vi "Calculate Pixel Reciprocals.vi"(11 "Sorted Triangle":T1={"Top Vertex"={"Position"={"x"=0.0, "y"=0.0, "z"=0.0}, "UV"={"u"=0.0, "v"=0.0}, "Colour"=12517256}, "Mid Vertex"={"Position"={"x"=0.0, "y"=0.0, "z"=0.0}, "UV"={"u"=0.0, "v"=0.0}, "Colour"=12517256}, "Bottom Vertex"={"Position"={"x"=0.0, "y"=0.0, "z"=0.0}, "UV"={"u"=0.0, "v"=0.0}, "Colour"=12517256}, "Alpha"=0.0, "Alpha Blending Enabled"=FALSE, "Colour"=0, "Material"={"Diffuse Colour"=0, "Texture"={"Pixels"=refnum, "Size"={"Width"=0, "Height"=0}}}} {"Bottom Vertex"."UV"."v" min=0 max=1 step=0.1; "Bottom Vertex"."UV"."u" min=0 max=1 step=0.1; "Mid Vertex"."UV"."v" min=0 max=1 step=0.1; "Mid Vertex"."UV"."u" min=0 max=1 step=0.1; "Top Vertex"."UV"."v" min=0 max=1 step=0.1; "Top Vertex"."UV"."u" min=0 max=1 step=0.1}) -> (3 "Columns Pixels Per Row":T8)   [LabVIEW 2020, in "Raster (FPGA).lvlib"]
uses:
  Raster (FPGA).lvlib
  Reciprocals.ctl
  Libraries/3D/Vector 3D.ctl
  Libraries/3D/3D.lvlib
  Libraries/3D/Vertex.ctl
  Libraries/3D/Triangle (Sorted).ctl
  Libraries/3D/Material.ctl
  Libraries/Raster/UV.ctl
  Libraries/Raster/Raster.lvlib
  Libraries/Raster/Rectangle Dimensions.ctl
  Libraries/Raster/Texture.ctl
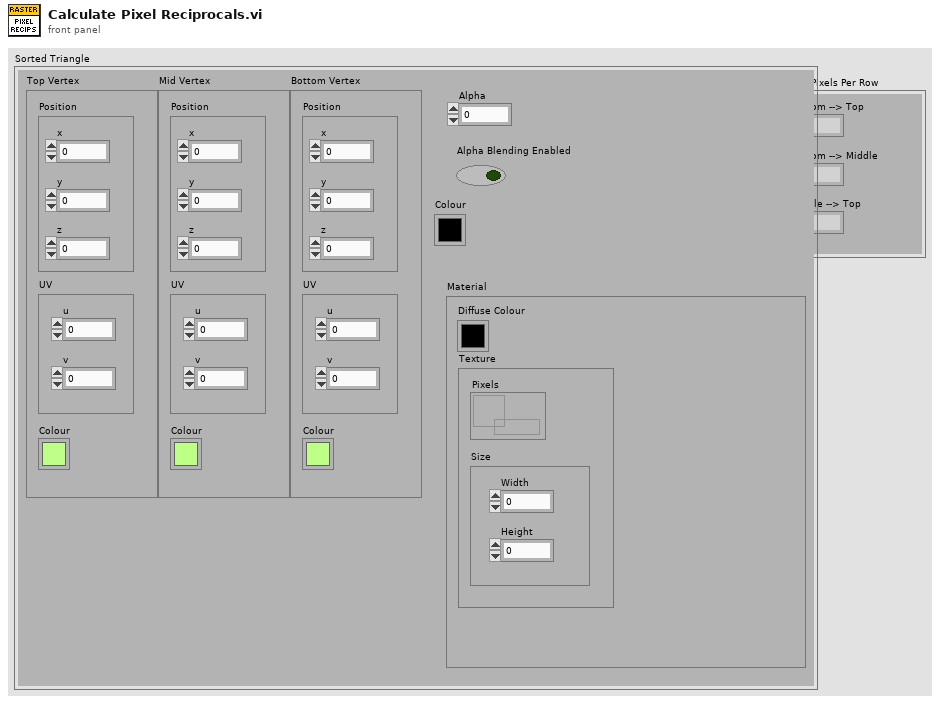
[diagram p1: front panel]
types:
  T1 = typedef "3D.lvlib/Triangle (Sorted).ctl" = cluster{"Top Vertex":T2, "Mid Vertex":T2, "Bottom Vertex":T2, "Alpha":dbl, "Alpha Blending Enabled":bool, "Colour":u32, "Material":T5}
  T2 = typedef "3D.lvlib/Vertex.ctl" = cluster{"Position":T3, "UV":T4, "Colour":u32}
  T3 = typedef "3D.lvlib/Vector 3D.ctl" = cluster{"x":sgl, "y":sgl, "z":sgl}
  T4 = typedef "Raster.lvlib/UV.ctl" = cluster{"u":sgl, "v":sgl}
  T5 = typedef "3D.lvlib/Material.ctl" = cluster{"Diffuse Colour":u32, "Texture":T6}
  T6 = typedef "Raster.lvlib/Texture.ctl" = cluster{"Pixels":refnum<data-value>, "Size":T7}
  T7 = typedef "Raster.lvlib/Rectangle Dimensions.ctl" = cluster{"Width":u32, "Height":u32}
  T8 = typedef "Raster (FPGA).lvlib/Reciprocals.ctl" = cluster{"Bottom --> Top":sgl, "Bottom --> Middle":sgl, "Middle --> Top":sgl}
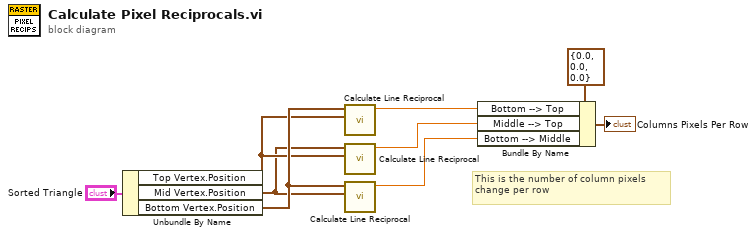
[diagram p0: block diagram]
diagram:
  # "This is the number of column pixels change per row"
  n1 = Unbundle By Name("Sorted Triangle") -> ("Top Vertex.Position"=w2:T3, "Mid Vertex.Position"=w1:T3, "Bottom Vertex.Position"=w3:T3)
  n2 = call "Calculate Line Reciprocal.vi"("P2"=w2, "P1"=w3) -> ("Column Pixels Per Row"=w5:sgl)  [unwired: 9 in]
  n3 = call "Calculate Line Reciprocal.vi"("P2"=w2, "P1"=w1) -> ("Column Pixels Per Row"=w6:sgl)  [unwired: 9 in]
  n4 = call "Calculate Line Reciprocal.vi"("P2"=w1, "P1"=w3) -> ("Column Pixels Per Row"=w7:sgl)  [unwired: 9 in]
  n5 = Bundle By Name(cluster=T8 {"Bottom --> Top"=0.0, "Bottom --> Middle"=0.0, "Middle --> Top"=0.0} ("Reciprocals"), "Bottom --> Top"=w5, "Middle --> Top"=w6, "Bottom --> Middle"=w7) -> (→"Columns Pixels Per Row":T8)
